vi "FrameSync.vi"(6 "LowTime":dbl=5e-06, 7 "Gate Length":dbl=0.09 format="%.6f", 11 "Main Digitizer":T1=enum."NI Digitizer") -> (0 "error out":errorcluster, 3 "task out":refnum<k21>)   [LabVIEW 2022 SP3]
uses:
  ScanningControl/Digitizers/-DigitizerRoutines/Digitizer.ctl
  <vilib>/DAQmx/configure/trigger.llb/DAQmx Start Trigger (Digital Edge).vi
  <resource>/objmgr/daqmx.rc
panel:
  # "CTR 6 of Timer gets used for Alazar.\nCTR 0 of Quantel Quant gets used if no Alazar\nAlazar has a frame grab trigger line so don't need external\nbox for frame synch."
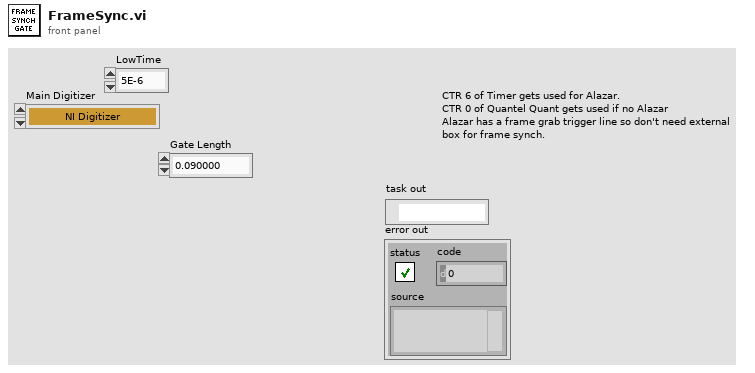
[diagram p1: front panel]
types:
  T1 = typedef "Digitizer.ctl" = enum16{"Acqiris Digitizer", "NI Digitizer", "LeCroy", "GaGe", "AlazarTech", "No Digitizer", "Teledyne"}
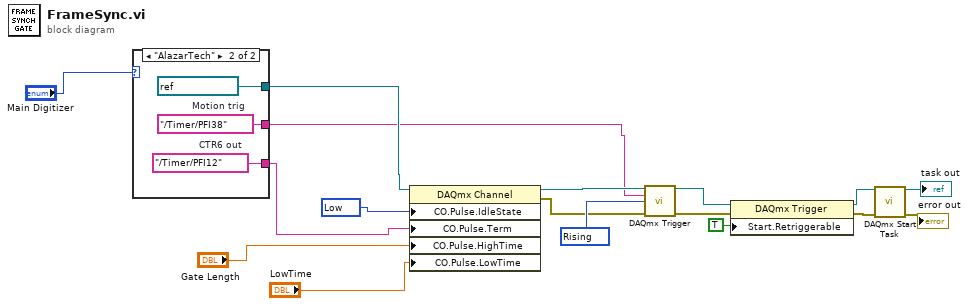
[diagram p0: block diagram]
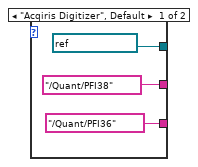
[diagram p2: hidden frame]
diagram:
  w6 = 10214 items=["High"=10192, "Low"=10214] ("CO.Pulse.IdleState")
  w14 = 10280 items=["Rising"=10280, "Falling"=10171] ("edge")
  n1 = case shown="\"AlazarTech\"" "Main Digitizer" {
    tunnel: [tag "/Quant/PFI36" ("OutputTerm") w23] -> w2
    tunnel: [tag "/Quant/PFI38" ("Gate") w22] -> w3
    tunnel: [refnum<k21> "QuantGate" ("task in") refnum<k21> "AvisoGate" ("task in")] -> w4
    frame "Acqiris Digitizer", Default {
    }
    frame "AlazarTech" {
      w23 = tag "/Timer/PFI12"  # CTR6 out
      w22 = tag "/Timer/PFI38"  # Motion trig
    }
  }
  n2 = property class="DAQmx Channel"(reference=w4, "CO.Pulse.IdleState"=w6, "CO.Pulse.Term"=w2, "CO.Pulse.HighTime"="Gate Length", "CO.Pulse.LowTime"="LowTime") -> (reference out=w11:refnum<k21>, error out=w10:errorcluster)  [unwired: 1 in]
  n3 = call-poly <vilib>:"DAQmx Trigger.vi"("task/channels in"=w11, "source"=w3, "edge"=w14, "error in"=w10) -> ("task out"=w13:refnum<k21>, "error out"=w12:errorcluster)  [unwired: 10 in]
  n4 = property class="DAQmx Trigger"(reference=w13, error in=w12, "Start.Retriggerable"=TRUE) -> (reference out=w17:refnum<k21>, error out=w16:errorcluster)
  n5 = call <vilib>:"DAQmx Start Task.vi"("task/channels in"=w17, "error in"=w16) -> ("task out"=→"task out":refnum<k21>, "error out"=→"error out":errorcluster)  [unwired: 12 in]
